vi "Circle.vi"(0 "Circle in":refnum<class "Circle.lvclass">, 1 "id":i32, 2 "x":i32, 3 "y":i32, 4 "radius":i32, 5 "error in (no error)":errorcluster) -> (14 "Circle out":refnum<class "Circle.lvclass">, 19 "error out":errorcluster)   [LabVIEW 2018, in "Circle.lvclass"]
uses:
  Circle.lvclass
  Circle.lvclass/Circle.ctl
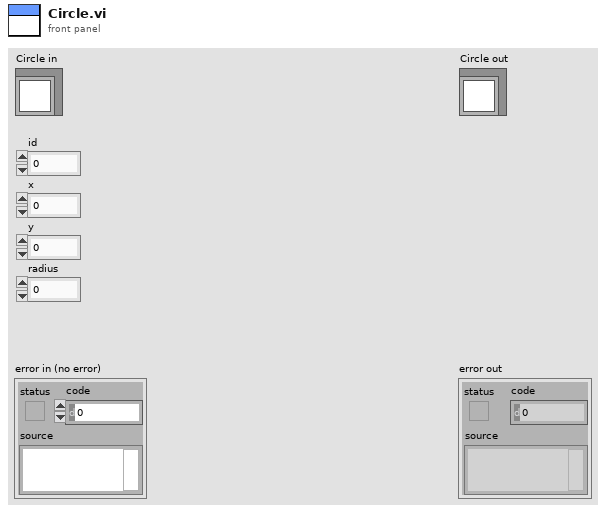
[diagram p1: front panel]
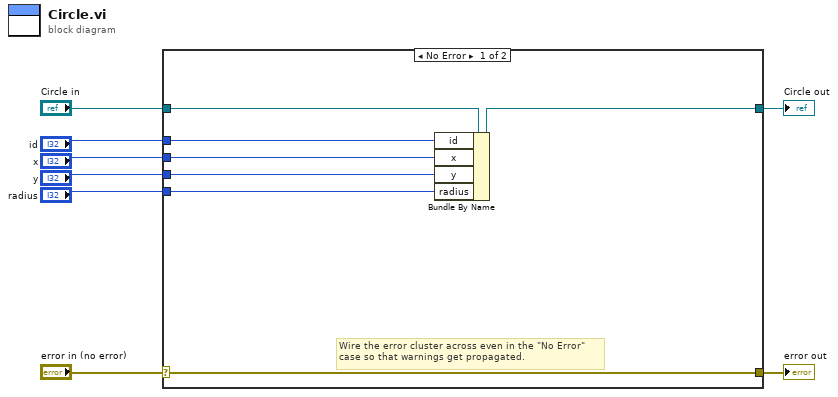
[diagram p0: block diagram]
diagram:
  n1 = case shown="No Error" "error in (no error)" {
    selector: "error in (no error)" -> [w14 w17]
    tunnel: [w14 w17] -> w7
    tunnel: [w13 w16] -> w5
    tunnel: "Circle in" -> [w15 w16]
    tunnel: "id" -> [w12 _]
    tunnel: "x" -> [w11 _]
    tunnel: "y" -> [w10 _]
    tunnel: "radius" -> [w9 _]
    frame No Error {
      # "Wire the error cluster across even in the \"No Error\"\ncase so that warnings get propagated."
      n2 = Bundle By Name(cluster=w15, "id"=w12, "x"=w11, "y"=w10, "radius"=w9) -> (w13:refnum<class "Circle.lvclass">)
    }
    frame Error {
    }
  }
  "error out" <- w7
  "Circle out" <- w5
